vi "Clear Array of Specific Errors.vi"(8 "error in":errorcluster, 11 "Error Codes":i32[](array[numeric])) -> (0 "error out":errorcluster)   [LabVIEW 2019, in "TSC Error.lvlib"]
doc: "This VI will clear a the error cluster if any in the array are on the error input.\n\nInputs:\n-Error Codes [array of I32] - the error codes to compare to and clear if it is the existing error\n-error in\n\nOutputs:\n-error out\n\n<b>Code Developed By:</b>\nDaniel Coons\nTechnology Service Corporation\n1983 S Liberty Drive\nBloomington, IN 47403\nwww.tsc.com/atcs"
uses:
  TSC Error.lvlib
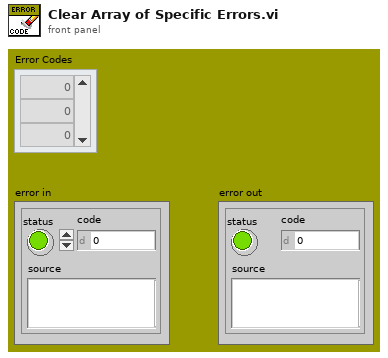
[diagram p1: front panel]
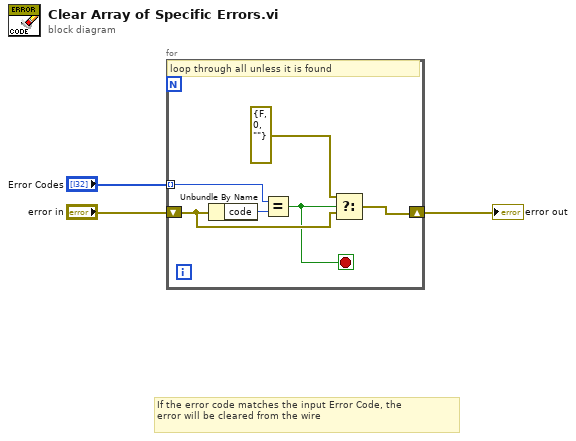
[diagram p0: block diagram]
diagram:
  # "If the error code matches the input Error Code, the \nerror will be cleared from the wire"
  n1 = for {
    shift-right: [w8] -> w2
    shift-left: "error in" -> [w9]
    tunnel: "Error Codes" -> [w5] mode=indexing
    stop <- w4 stop-if-true
    # "loop through all unless it is found"
    n2 = Unbundle By Name(w9) -> ("code"=w7:i32)
    n3 = Equal?(x=w5, y=w7) -> (x = y?=w4:bool)
    n4 = Select(t=errorcluster {"status"=FALSE, "code"=0, "source"=""}, s=w4, f=w9) -> (s? t:f=w8:errorcluster)
  }
  "error out" <- w2
